vi "Creators Status Created Queues.vi"(11 "Template Event in":refnum<class "Template Event.lvclass">) -> (0 "Created Queue Count":i32, 1 "Created Queue Aliases":string[](array[string]), 2 "Created Queue Exist?":bool, 3 "Template Event out":refnum<class "Template Event.lvclass">)   [LabVIEW 2021, in "_Template.lvlib" / "Templates.lvlib" / "Template Event.lvlib" / "Template Event.lvclass"]
uses:
  Template Event.lvclass
  Template Event.lvclass/Template Event.ctl
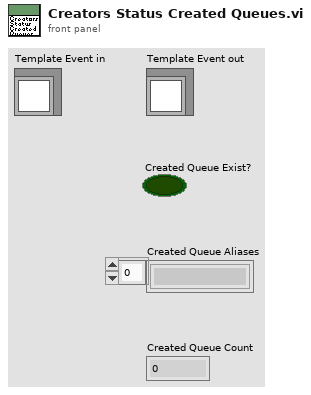
[diagram p1: front panel]
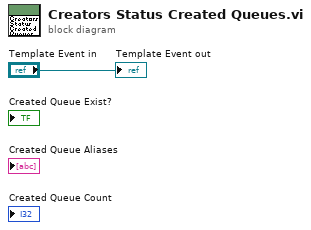
[diagram p0: block diagram]
diagram:
  "Template Event out" <- "Template Event in"
